vi "FIle_Create If Needed.vi"(8 "error in (no error)":errorcluster, 11 "dup path in":path) -> (0 "error out":errorcluster, 2 "file or folder exists?":bool, 3 "dup path out":path)   [LabVIEW 2020]
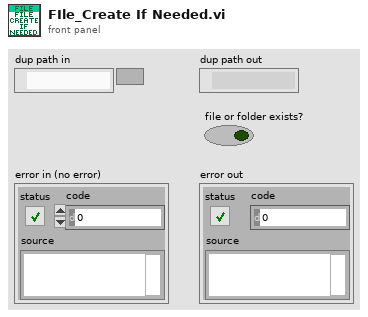
[diagram p1: front panel]
types:
  T1 = enum16{"open", "replace", "create", "open or create", "replace or create", "replace or create with confirmation"}
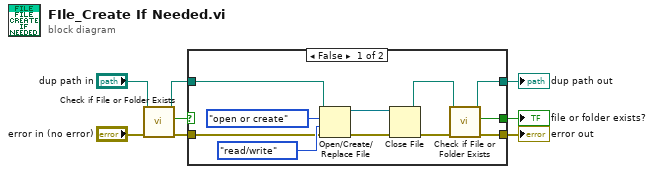
[diagram p0: block diagram]
diagram:
  n1 = call <vilib>:"Check if File or Folder Exists.vi"("error in (no error)"="error in (no error)", "path"="dup path in") -> ("error out"=w1:errorcluster, "file or folder exists?"=w3:bool, "dup path"=w4:path)  [unwired: 7 in]
  n2 = case shown="False" w3 {
    selector: w3 -> [_ w21]
    tunnel: [w19 w22] -> w8
    tunnel: [w13 w21] -> w7
    tunnel: [w12 w20] -> w6
    tunnel: w1 -> [w10 w22]
    tunnel: w4 -> [w9 w20]
    frame False {
      n3 = Open/Create/Replace File(file path (use dialog)=w9, error in=w10, operation (0:open)=T1."open or create", access (0:read/write)=enum16{"read/write", "read-only", "write-only"}."read/write") -> (refnum out=w11:refnum<file>, error out=w17:errorcluster)  [unwired: 2 in, 1 out]
      n4 = Close File(refnum=w11, error in=w17) -> (path=w16:path, error out=w18:errorcluster)
      n5 = call <vilib>:"Check if File or Folder Exists.vi"("error in (no error)"=w18, "path"=w16) -> ("error out"=w19:errorcluster, "file or folder exists?"=w13:bool, "dup path"=w12:path)  [unwired: 7 in]
    }
    frame True {
    }
  }
  "error out" <- w8
  "file or folder exists?" <- w7
  "dup path out" <- w6
